vi "Get Ref Prop.vi"(8 "error in (no error)":errorcluster, 11 "SequenceFile in":refnum<class "SequenceFile.lvclass">) -> (0 "error out":errorcluster, 2 "Ref":refnum<k7>, 3 "SequenceFile out":refnum<class "SequenceFile.lvclass">)   [LabVIEW 2019, in "HTS.lvlib" / "SequenceFile.lvclass"]
uses:
  SequenceFile.lvclass
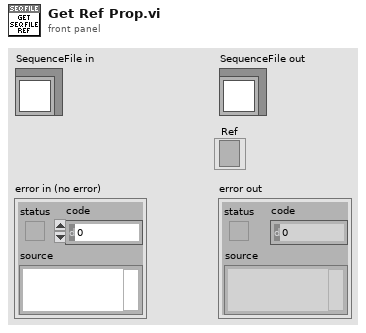
[diagram p1: front panel]
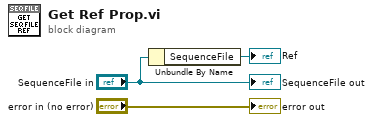
[diagram p0: block diagram]
diagram:
  n1 = Unbundle By Name("SequenceFile in") -> ("SequenceFile"=→"Ref":refnum<k7>)
  "error out" <- "error in (no error)"
  "SequenceFile out" <- "SequenceFile in"
